vi "Database.File.Find.vi"(8 "error in (no error)":errorcluster) -> (0 "error out":errorcluster, 2 "FileName":string)   [LabVIEW 2016]
uses:
  Global/ApplicationGlobal.vi
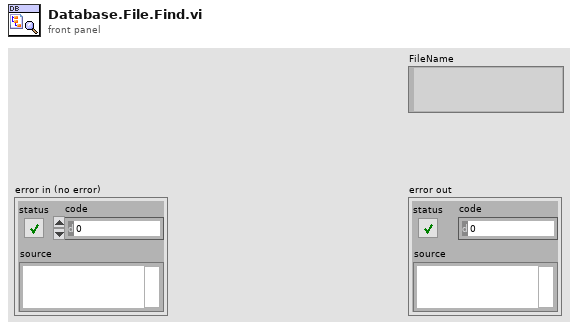
[diagram p1: front panel]
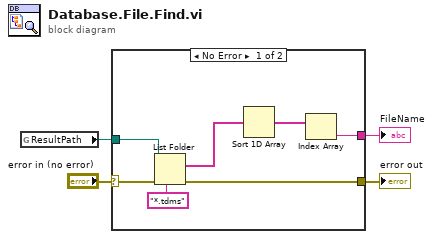
[diagram p0: block diagram]
diagram:
  n1 = global read "ApplicationGlobal.vi" "ResultPath"() -> (w2:path)
  n2 = case shown="No Error" "error in (no error)" {
    selector: "error in (no error)" -> [w11 w12]
    tunnel: [w5 w12] -> w4
    tunnel: w2 -> [w9 _]
    tunnel: [w6 _] -> w1
    frame No Error {
      n3 = List Folder(path=w9, pattern="*.tdms", error in=w11) -> (filenames=w8:string[], error out=w5:errorcluster)  [unwired: 1 in, 2 out]
      n4 = Sort 1D Array(array=w8) -> (sorted array=w7:string[])
      n5 = Index Array(array=w7) -> (element=w6:string)  [unwired: 1 in]
    }
    frame Error {
    }
  }
  "error out" <- w4
  "FileName" <- w1
